vi "RegisterColumnIDs.vi"(2 "Column IDs":u32[](array[numeric]), 3 "Display Names":string[](array[string]), 4 "kSAComm ref in":refnum<k24>) -> (0 "Success":bool, 1 "kSAComm ref out":refnum<k24>)   [LabVIEW 2019]
uses:
  C:/Users/tim/Documents/kSAComm LabView Sample/kSACommInterface.dll
  kSACommInterface.dll
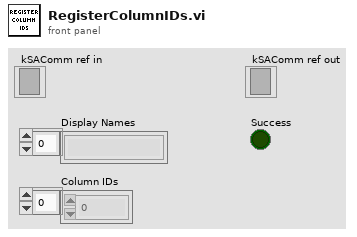
[diagram p1: front panel]
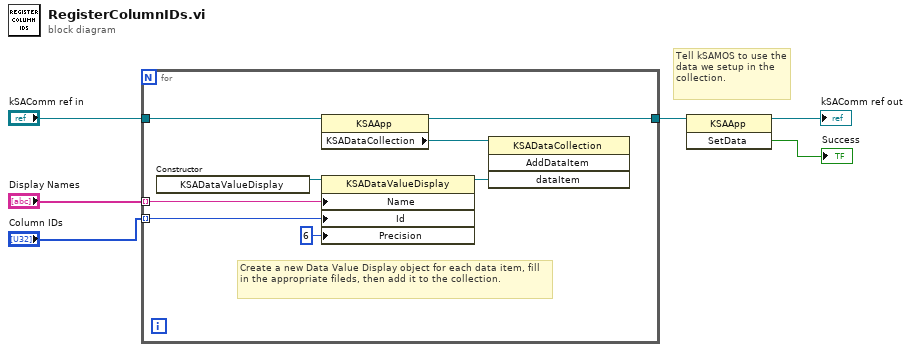
[diagram p0: block diagram]
diagram:
  # "Tell kSAMOS to use the data we setup in the collection."
  n1 = for {
    tunnel: "kSAComm ref in" -> [w14]
    tunnel: "Display Names" -> [w13] mode=indexing
    tunnel: "Column IDs" -> [w12] mode=indexing
    tunnel: [w8] -> w6
    # "Create a new Data Value Display object for each data item, fill in the appropriate fileds, then add it to the collection."
    n2 = constructor class="KSADataValueDisplay"() -> (reference out=w9:refnum<k24>)  [unwired: 3 in, 2 out]
    n3 = property class="KSAApp"(reference=w14) -> (reference out=w8:refnum<k24>, "KSADataCollection"=w11:refnum<k24>)  [unwired: 1 in, 1 out]
    n4 = property class="KSADataValueDisplay"(reference=w9, "Name"=w13, "Id"=w12, "Precision"=6) -> (reference out=w10:refnum<k24>)  [unwired: 1 in, 1 out]
    n5 = invoke class="KSADataCollection" method="AddDataItem"(reference=w11, "dataItem"=w10) -> ()  [unwired: 2 in, 4 out]
  }
  n6 = invoke class="KSAApp" method="SetData"(reference=w6) -> (reference out=→"kSAComm ref out":refnum<k24>, "SetData"=→"Success":bool)  [unwired: 2 in, 1 out]
